vi "GSET_VIDesactivationEventRef.vi"(7 "Action":enum16{"Get", "Set"}(ring)=enum."Set", 8 "error in (no error)":errorcluster, 10 "VIDesactivationEvent in":refnum<user-event>, 11 "VI Activation in":refnum<class "VIActivation.lvclass">) -> (0 "error out":errorcluster, 2 "VIDesactivationEvent out":refnum<user-event>, 3 "VI Activation out":refnum<class "VIActivation.lvclass">)   [LabVIEW 2021, in "VIActivation.lvlib" / "VIActivation.lvclass"]
uses:
  VIActivation.lvclass
  VIActivationEvents.ctl
  VIActivation.lvclass/VIActivation.ctl
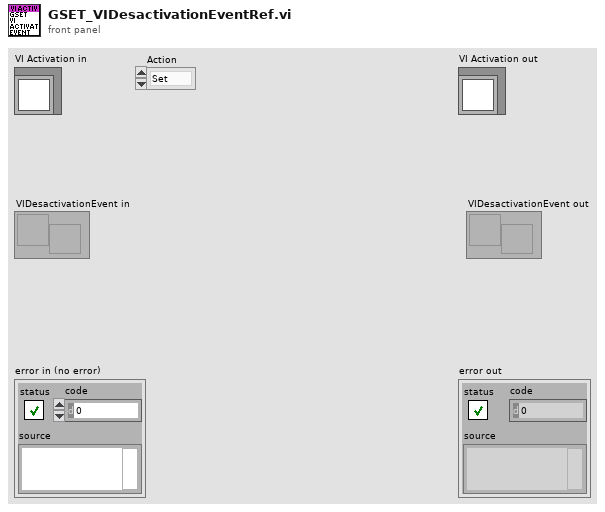
[diagram p1: front panel]
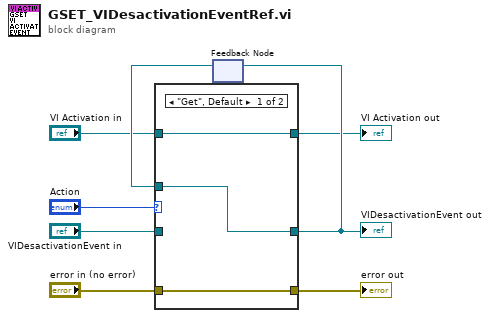
[diagram p0: block diagram]
diagram:
  n1 = feedback #1() -> (w6:refnum<user-event>)  [unwired: 1 in]
  n2 = case shown="\"Get\", Default" "Action" {
    tunnel: "VIDesactivationEvent in" -> [_ w14]
    tunnel: [w11 w14] -> w7
    tunnel: w6 -> [w11 _]
    tunnel: "error in (no error)" -> [w10 w13]
    tunnel: [w10 w13] -> w3
    tunnel: "VI Activation in" -> [w9 w12]
    tunnel: [w9 w12] -> w1
    frame "Get", Default {
    }
    frame "Set" {
    }
  }
  "error out" <- w3
  "VI Activation out" <- w1
  "VIDesactivationEvent out" <- w7
  n3 = feedback-in #1(w7) -> ()
